vi "Sendfilepath.vi"(8 "error in (no error)":errorcluster, 9 "String":string, 10 "base path":path, 11 "VI in":refnum<vi>) -> (0 "error out":errorcluster, 3 "VI out":refnum<vi>)   [LabVIEW 2015]
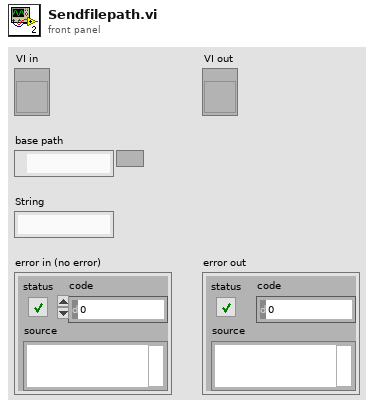
[diagram p1: front panel]
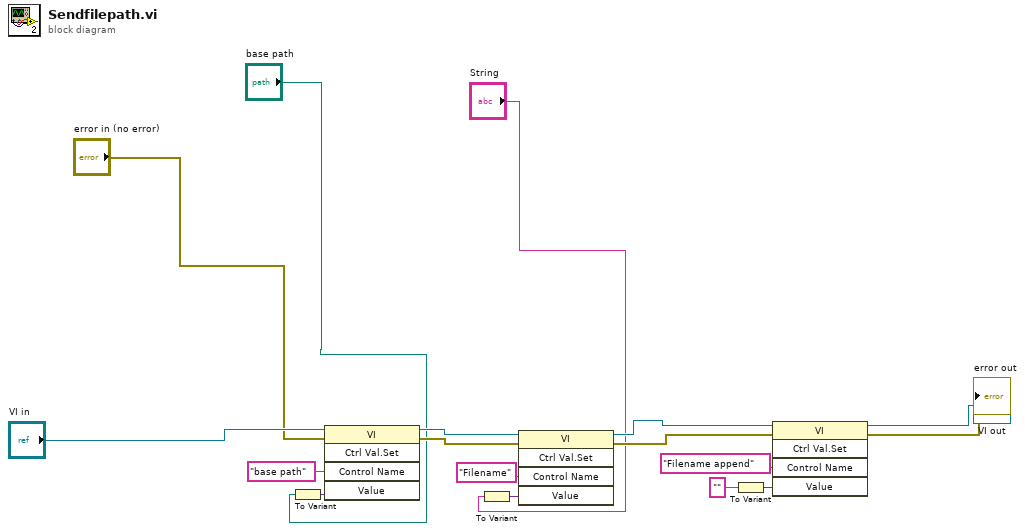
[diagram p0: block diagram]
diagram:
  n1 = To Variant(anything="base path") -> (Variant=w12:variant)
  n2 = invoke class="VI" method="Ctrl Val.Set"(reference="VI in", error in="error in (no error)", "Control Name"="base path", "Value"=w12) -> (reference out=w7:refnum<vi>, error out=w8:errorcluster)  [unwired: 1 in, 3 out]
  n3 = To Variant(anything="String") -> (Variant=w10:variant)
  n4 = invoke class="VI" method="Ctrl Val.Set"(reference=w7, error in=w8, "Control Name"="Filename", "Value"=w10) -> (reference out=w16:refnum<vi>, error out=w17:errorcluster)  [unwired: 1 in, 3 out]
  n5 = To Variant(anything="") -> (Variant=w15:variant)
  n6 = invoke class="VI" method="Ctrl Val.Set"(reference=w16, error in=w17, "Control Name"="Filename append", "Value"=w15) -> (reference out=→"VI out":refnum<vi>, error out=→"error out":errorcluster)  [unwired: 1 in, 3 out]
